vi "example_00_excessive_data.vi"() -> ()   [LabVIEW 2015, in "lv-graph.lvlib"]
doc: "This is a simple example showing how graph's have a memory limitation: you can put more data into memory if you DON'T put it into a graph. Setting data_into_graph to true should generally FAIL causing the VI to crash, but if you don't put it into the graph, you'll see that you can view all of the data as long as you navigate it using the scrollbar."
uses:
  advanced/build_graph-single_axis.vi
  lv-graph.lvlib
panel:
  in  "clear_graph":bool
  in  "data_into_graph":bool=TRUE
  in  "stop":bool
  in  "scrollbar":i32(c297)
  out "graph":T1(graph)
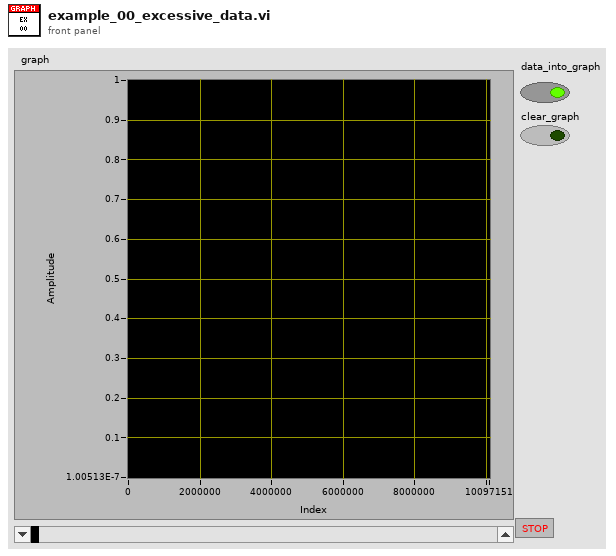
[diagram p1: front panel]
types:
  T1 = cluster{"Time [] out":dbl[], "Data[][] out":dbl[]}[]
  T2 = cluster{"x_scale_maximum":dbl, "x_scale_minimum":dbl, "y_scale_maximum":dbl, "y_scale_minimum":dbl}
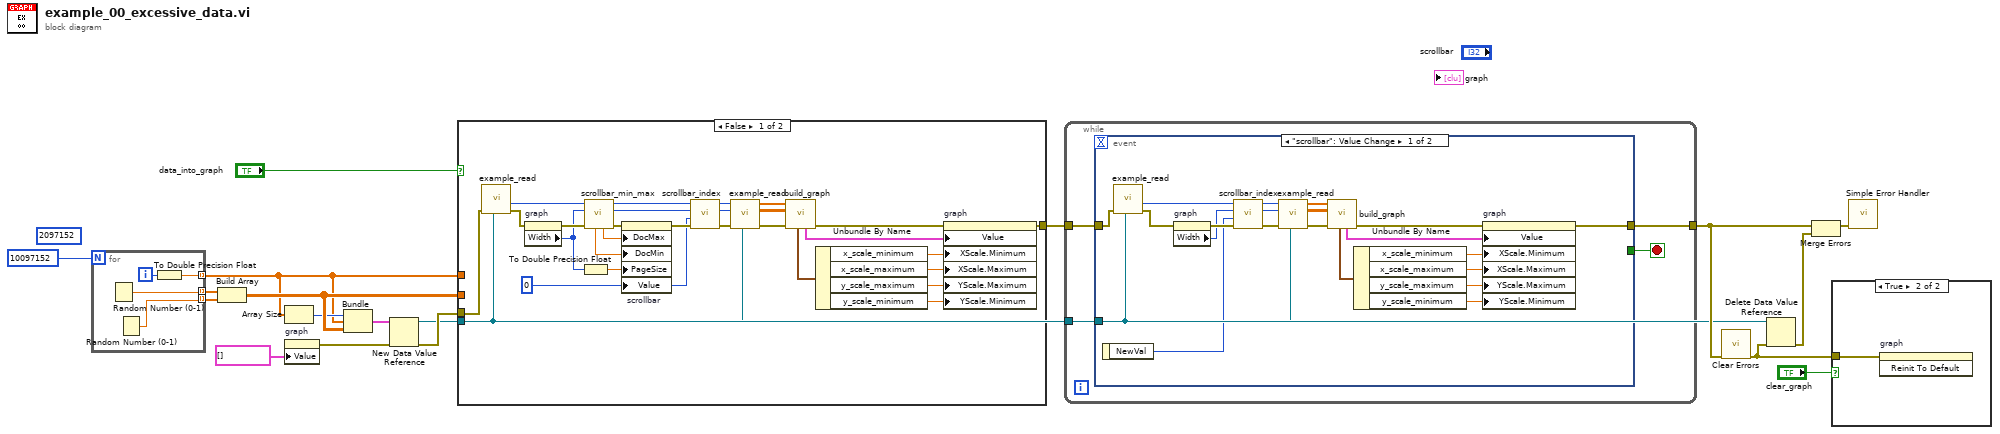
[diagram p0: block diagram]
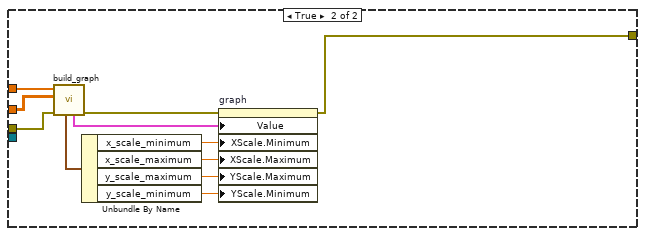
[diagram p3: hidden frame]
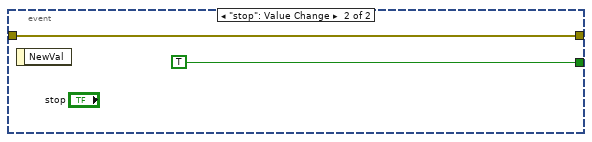
[diagram p4: hidden frame]
diagram:
  (unwired) 2097152
  n1 = for {
    N: 10097152 ("points_to_generate") -> [_]
    tunnel: [w21] -> w8 mode=indexing
    tunnel: [w20] -> w14 mode=indexing
    tunnel: [w19] -> w13 mode=indexing
    i -> [w22]
    n2 = Random Number (0-1)() -> (number: 0 to 1=w20:dbl)
    n3 = Random Number (0-1)() -> (number: 0 to 1=w19:dbl)
    n4 = To Double Precision Float(number=w22) -> (double precision float=w21:dbl)
  }
  n5 = Build Array(w14, w13) -> (w10:dbl[][])
  n6 = Array Size(array=w8) -> (size(s)=w9:i32)
  n7 = property on="graph" class="XYGraph (strict)"("Value"=T1 [] ("Graph")) -> (error out=w12:errorcluster)  [unwired: 2 in, 1 out]
  n8 = Bundle(w9, w8, w10) -> (w7:cluster{i32, dbl[], dbl[][]})  [unwired: 1 in]
  n9 = New Data Value Reference(data value=w7, error in=w12) -> (data value reference=w4:refnum<data-value>, error out=w11:errorcluster)
  n10 = case shown="False" "data_into_graph" {
    tunnel: [w24 w57] -> w3
    tunnel: w11 -> [w39 w59]
    tunnel: w10 -> [_ w55]
    tunnel: w8 -> [_ w56]
    tunnel: w4 -> [w25 _]
    frame False {
      w23 = 0 ("Scrollbar")
      n11 = call "example_read.vi"("dvr"=w25, "error in (no error)"=w39) -> ("error out"=w45:errorcluster, "index"=w34:i32)  [unwired: 6 in, 2 out]
      n12 = property on="graph" class="XYGraph (strict)"(error in=w45) -> (error out=w44:errorcluster, "Width"=w43:u32)  [unwired: 1 in, 1 out]
      n13 = To Double Precision Float(number=w43) -> (double precision float=w42:dbl)
      n14 = call "scrollbar_min_max.vi"("error in (no error)"=w44, "width_height"=w43, "data_index in"=w34) -> ("error out"=w46:errorcluster, "scrollbar_doc_max"=w37:dbl, "scrollbar_doc_min"=w38:dbl)  [unwired: 6 in]
      n15 = property on="scrollbar" class="Scroll (strict)"(error in=w46, "DocMax"=w37, "DocMin"=w38, "PageSize"=w42, "Value"=w23) -> (error out=w47:errorcluster)  [unwired: 1 in, 1 out]
      n16 = call "scrollbar_index.vi"("error in (no error)"=w47, "seek"=w23, "width_height"=w43, "data_available"=w34) -> ("error out"=w41:errorcluster, "length"=w32:i32, "index"=w33:i32)  [unwired: 5 in]
      n17 = call "example_read.vi"("dvr"=w25, "error in (no error)"=w41, "length"=w32, "index in"=w33) -> ("error out"=w40:errorcluster, "y_axis"=w35:dbl[][], "x_axis"=w36:dbl[])  [unwired: 4 in, 1 out]
      n18 = call-poly "build_graph.vi"("error in (no error)"=w40, "y_axis"=w35, "x_axis"=w36) -> ("error out"=w48:errorcluster, "graph_data"=w30:cluster{dbl[], dbl[]}[], "scale_ranges"=w31:T2)  [unwired: 6 in]
      n19 = Unbundle By Name(w31) -> ("x_scale_minimum"=w29:dbl, "x_scale_maximum"=w28:dbl, "y_scale_maximum"=w27:dbl, "y_scale_minimum"=w26:dbl)
      n20 = property on="graph" class="XYGraph (strict)"(error in=w48, "Value"=w30, "XScale.Minimum"=w29, "XScale.Maximum"=w28, "YScale.Maximum"=w27, "YScale.Minimum"=w26) -> (error out=w24:errorcluster)  [unwired: 1 in, 1 out]
    }
    frame True {
      n21 = call-poly "build_graph.vi"("error in (no error)"=w59, "y_axis"=w55, "x_axis"=w56) -> ("error out"=w58:errorcluster, "graph_data"=w53:cluster{dbl[], dbl[]}[], "scale_ranges"=w54:T2)  [unwired: 6 in]
      n22 = Unbundle By Name(w54) -> ("x_scale_minimum"=w52:dbl, "x_scale_maximum"=w51:dbl, "y_scale_maximum"=w50:dbl, "y_scale_minimum"=w49:dbl)
      n23 = property on="graph" class="XYGraph (strict)"(error in=w58, "Value"=w53, "XScale.Minimum"=w52, "XScale.Maximum"=w51, "YScale.Maximum"=w50, "YScale.Minimum"=w49) -> (error out=w57:errorcluster)  [unwired: 1 in, 1 out]
    }
  }
  n24 = while {
    tunnel: w3 -> [w63]
    tunnel: [w61] -> w18
    tunnel: w4 -> [w60]
    stop <- w62 stop-if-true
    n25 = event shown="[0] \"scrollbar\": Value Change" {
      selector: _ -> [_ _]
      dyn-events: _ -> [_ _]
      timeout: _ -> [_ _]
      tunnel: w63 -> [w80 w85]
      tunnel: [_ TRUE] -> w62
      tunnel: [w79 w85] -> w61
      tunnel: w60 -> [w67 _]
      event "scrollbar": Value Change {
        n26 = event-data() -> ("NewVal"=w64:i32)  [unwired: 1 in]
        n27 = call "example_read.vi"("dvr"=w67, "error in (no error)"=w80) -> ("error out"=w81:errorcluster, "index"=w76:i32)  [unwired: 6 in, 2 out]
        n28 = property on="graph" class="XYGraph (strict)"(error in=w81) -> (error out=w84:errorcluster, "Width"=w82:u32)  [unwired: 1 in, 1 out]
        n29 = call "scrollbar_index.vi"("error in (no error)"=w84, "seek"=w64, "width_height"=w82, "data_available"=w76) -> ("error out"=w78:errorcluster, "length"=w68:i32, "index"=w69:i32)  [unwired: 5 in]
        n30 = call "example_read.vi"("dvr"=w67, "error in (no error)"=w78, "length"=w68, "index in"=w69) -> ("error out"=w77:errorcluster, "y_axis"=w65:dbl[][], "x_axis"=w66:dbl[])  [unwired: 4 in, 1 out]
        n31 = call-poly "build_graph.vi"("error in (no error)"=w77, "y_axis"=w65, "x_axis"=w66) -> ("error out"=w83:errorcluster, "graph_data"=w75:cluster{dbl[], dbl[]}[], "scale_ranges"=w74:T2)  [unwired: 6 in]
        n32 = Unbundle By Name(w74) -> ("x_scale_minimum"=w70:dbl, "x_scale_maximum"=w71:dbl, "y_scale_maximum"=w72:dbl, "y_scale_minimum"=w73:dbl)
        n33 = property on="graph" class="XYGraph (strict)"(error in=w83, "Value"=w75, "XScale.Minimum"=w70, "XScale.Maximum"=w71, "YScale.Maximum"=w72, "YScale.Minimum"=w73) -> (error out=w79:errorcluster)  [unwired: 1 in, 1 out]
      }
      event "stop": Value Change {
        n34 = event-data() -> ()  [unwired: 1 in, 1 out]
      }
    }
  }
  n35 = call <vilib>:"Clear Errors.vi"("error in (no error)"=w18) -> ("error out"=w2:errorcluster)  [unwired: 5 in, 1 out]
  n36 = Delete Data Value Reference(data value reference=w4, error in=w2) -> (error out=w5:errorcluster)  [unwired: 1 out]
  n37 = Merge Errors(w18, w5) -> (w6:errorcluster)
  n38 = case shown="True" "clear_graph" {
    tunnel: w2 -> [_ w87]
    frame False {
    }
    frame True {
      n39 = invoke on="graph" class="XYGraph (strict)" method="Reinit To Default"(error in=w87) -> ()  [unwired: 2 in, 3 out]
    }
  }
  n40 = call <vilib>:"Simple Error Handler.vi"("error in (no error)"=w6) -> ()  [unwired: 4 in, 5 out]
